vi "Cache Cal Standard.vi"(0 "Cal Standard Base in":refnum<class "Cal Standard Base.lvclass">, 11 "error in (no error)":errorcluster) -> (4 "Cal Standard Base out":refnum<class "Cal Standard Base.lvclass">, 15 "error out":errorcluster)   [LabVIEW 2023, in "RFFixtureCharact.Instruments.lvlib" / "Cal Standard Factory.lvclass"]
uses:
  Cal Standard Factory/Cal Standard Factory.lvclass
  Cal Standard Base.lvclass
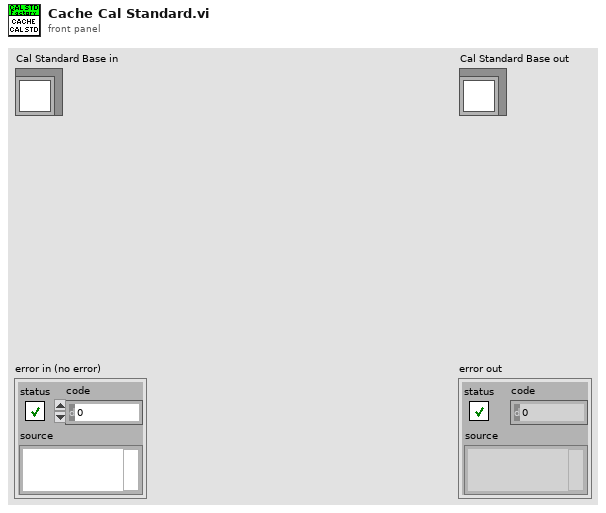
[diagram p1: front panel]
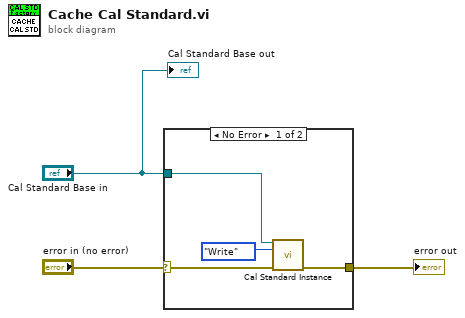
[diagram p0: block diagram]
diagram:
  n1 = case shown="No Error" "error in (no error)" {
    selector: "error in (no error)" -> [w7 w8]
    tunnel: [w6 w8] -> w2
    tunnel: "Cal Standard Base in" -> [w4 _]
    frame No Error {
      n2 = call "Cal Standard Instance.vi"("Cal Standard Base in"=w4, "Operation"=enum16{"Read", "Write", "Clear"}."Write", "error in (no error)"=w7) -> ("error out"=w6:errorcluster)  [unwired: 10 in, 2 out]
    }
    frame Error {
    }
  }
  "error out" <- w2
  "Cal Standard Base out" <- "Cal Standard Base in"
